vi "Ball ROI (SubVI).vi"(5 "ROI Descriptor COLOR Mask":T2={"Global Rectangle"=[109, 72, 345, 284], "Contours"=[{"ID"=enum."External", "Type"=3, "Coordinates"=[109, 72, 345, 284]}]} {"Contours"."Type" items=["No Selection", "Point", "Line", "Rectangle", "Oval", "Polygon", "Freehand Region", "Annulus", "Unused2", "Unused3", "Broken Line", "Freehand Line", "Rotated Rectangle"]}, 6 "divider (circle)":dbl=1.0, 8 "curY":dbl, 9 "curX":dbl, 10 "Boolean":bool, 11 "Digital in":refnum<vi>) -> (0 "x1":i32, 1 "y0":i32, 2 "x0":i32, 3 "ROI Descriptor COLOR Mask out":T2={"Global Rectangle"=[109, 72, 345, 284], "Contours"=[{"ID"=enum."External", "Type"=3, "Coordinates"=[109, 72, 345, 284]}]} {"Contours"."Type" items=["No Selection", "Point", "Line", "Rectangle", "Oval", "Polygon", "Freehand Region", "Annulus", "Unused2", "Unused3", "Broken Line", "Freehand Line", "Rotated Rectangle"]}, 4 "y1":i32)   [LabVIEW 2017]
panel:
  out "output cluster":T1
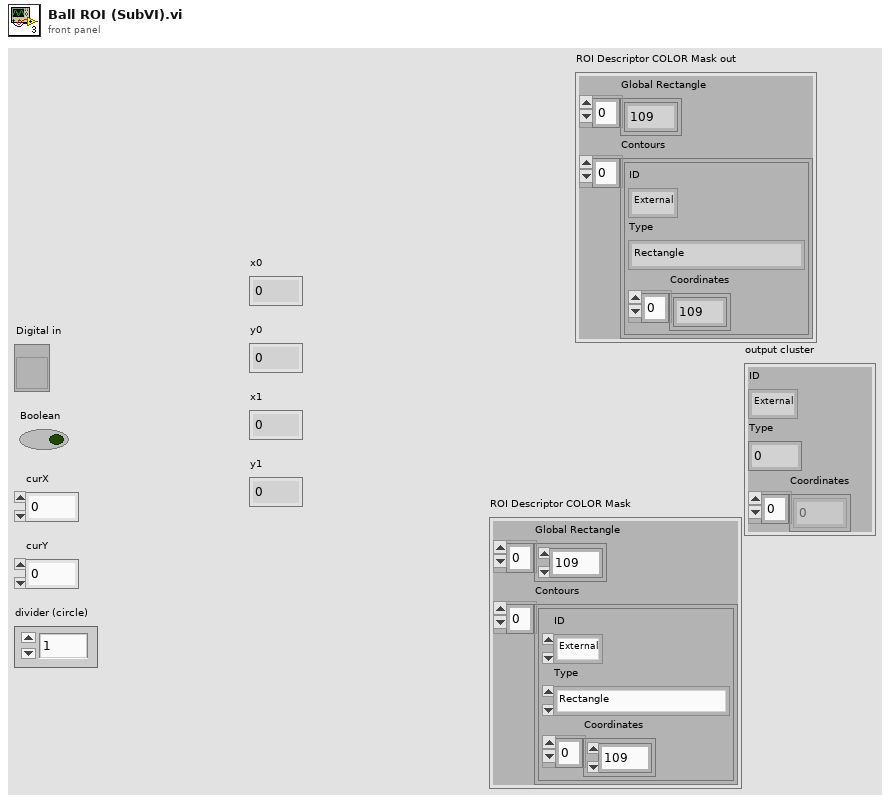
[diagram p1: front panel]
types:
  T1 = cluster{"ID":enum32{"External", "Internal"}, "Type":u32, "Coordinates":i32[]}
  T2 = cluster{"Global Rectangle":i32[], "Contours":cluster{"ID":enum32{"External", "Internal"}, "Type":u32, "Coordinates":i32[]}[]}
  T3 = cluster{"ID":enum32{"External", "Internal"}, "Type":u32, "Coordinates":i32[]}[]
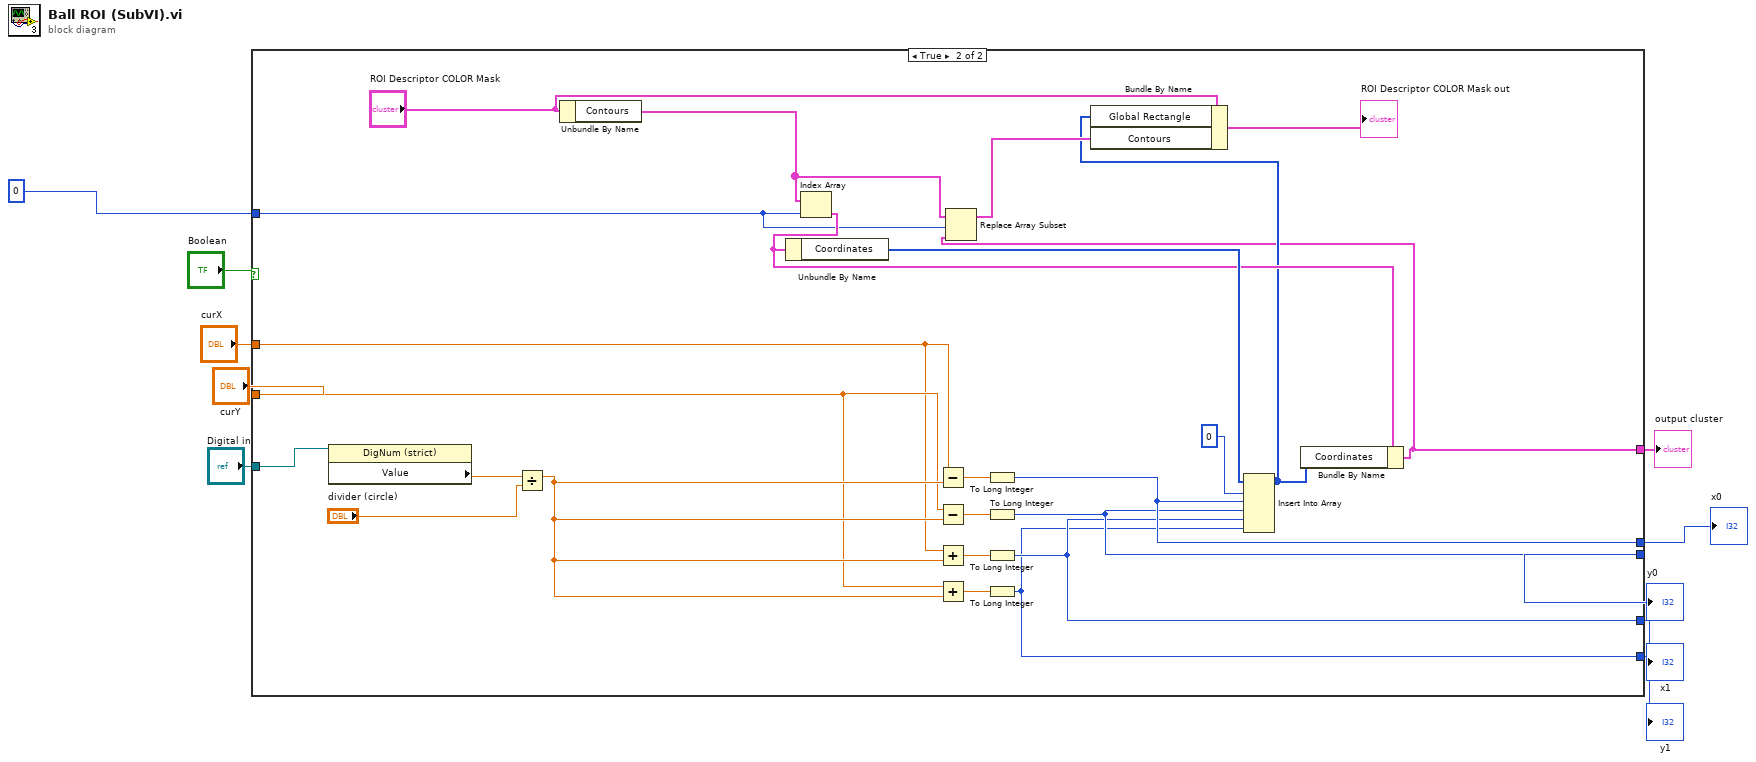
[diagram p0: block diagram]
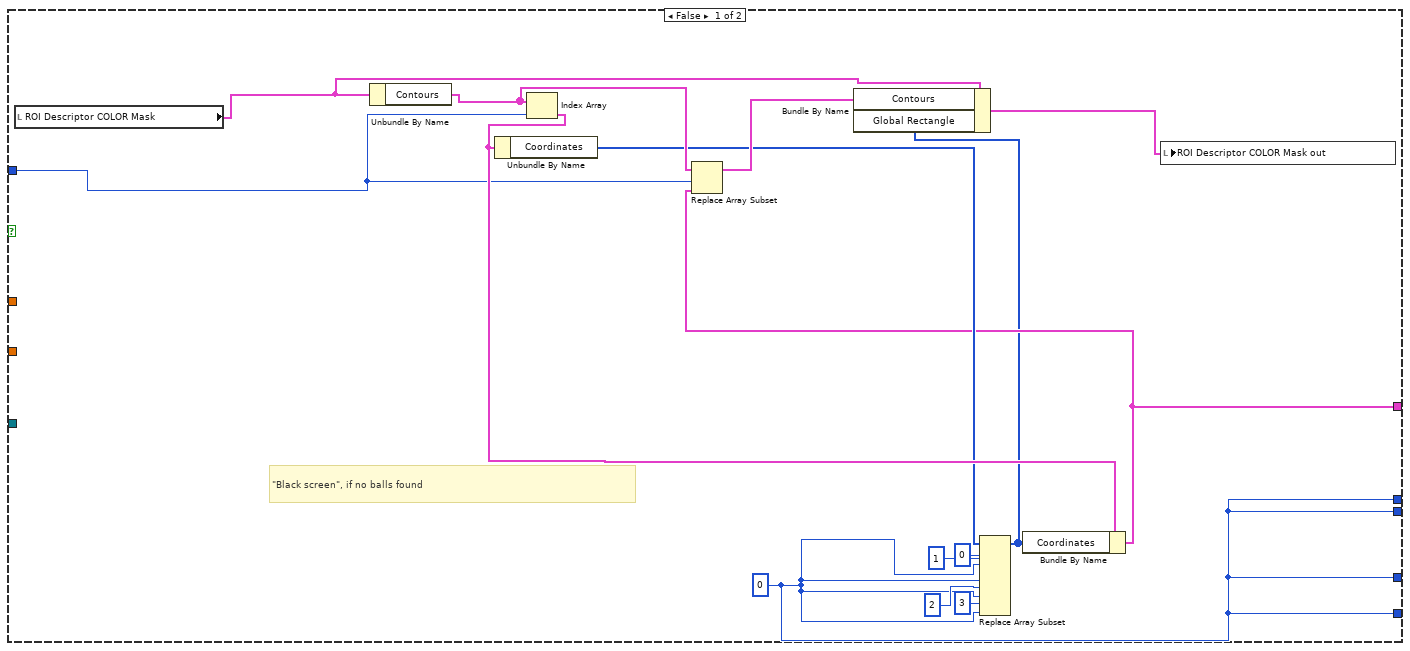
[diagram p2: hidden frame]
diagram:
  n1 = case shown="True" "Boolean" {
    tunnel: 0 ("Ball index") -> [w13 w27]
    tunnel: [w19 w30] -> w5
    tunnel: [w19 w31] -> w6
    tunnel: [w19 w33] -> w7
    tunnel: [w19 w32] -> w8
    tunnel: "curY" -> [_ w39]
    tunnel: "curX" -> [_ w38]
    tunnel: "Digital in" -> [_ w37]
    tunnel: [w12 w26] -> w1
    frame False {
      w19 = 0 ("index")
      # "\"Black screen\", if no balls found"
      n2 = local read "ROI Descriptor COLOR Mask"() -> (w15:T2)
      n3 = Unbundle By Name(w15) -> ("Contours"=w18:T3)
      n4 = Index Array(array=w18, index=w13) -> (element=w17:T1)
      n5 = Unbundle By Name(w17) -> ("Coordinates"=w16:i32[])
      n6 = Replace Array Subset(array=w16, new element #1=w19, index #1=0 ("index"), new element #2=w19, index #2=1 ("index"), new element #3=w19, index #3=2 ("index"), new element #4=w19, index #4=3 ("index")) -> (w11:i32[])
      n7 = Bundle By Name(cluster=w17, "Coordinates"=w11) -> (w12:T1)
      n8 = Replace Array Subset(array=w18, new element=w12, index=w13) -> (w20:T3)
      n9 = Bundle By Name(cluster=w15, "Contours"=w20, "Global Rectangle"=w11) -> (w14:T2)
      n10 = local write "ROI Descriptor COLOR Mask out"(w14) -> ()
    }
    frame True {
      n11 = property class="DigNum (strict)"(reference=w37) -> ("Value"=w40:dbl)  [unwired: 1 in, 2 out]
      n12 = Divide(x=w40, y="divider (circle)") -> (x/y=w44:dbl)
      n13 = Unbundle By Name("ROI Descriptor COLOR Mask") -> ("Contours"=w41:T3)
      n14 = Index Array(array=w41, index=w27) -> (element=w42:T1)
      n15 = Unbundle By Name(w42) -> ("Coordinates"=w43:i32[])
      n16 = Subtract(x=w38, y=w44) -> (x-y=w48:dbl)
      n17 = Subtract(x=w39, y=w44) -> (x-y=w47:dbl)
      n18 = Add(x=w38, y=w44) -> (x+y=w45:dbl)
      n19 = Add(x=w39, y=w44) -> (x+y=w46:dbl)
      n20 = To Long Integer(number=w48) -> (32bit integer=w33:i32)
      n21 = To Long Integer(number=w47) -> (32bit integer=w32:i32)
      n22 = To Long Integer(number=w45) -> (32bit integer=w31:i32)
      n23 = To Long Integer(number=w46) -> (32bit integer=w30:i32)
      n24 = Insert Into Array(array=w43, index=0, new element #1=w33, new element #2=w32, new element #3=w31, new element #4=w30) -> (w28:i32[])
      n25 = Bundle By Name(cluster=w42, "Coordinates"=w28) -> (w26:T1)
      n26 = Replace Array Subset(array=w41, new element=w26, index=w27) -> (w29:T3)
      n27 = Bundle By Name(cluster="ROI Descriptor COLOR Mask", "Global Rectangle"=w28, "Contours"=w29) -> (→"ROI Descriptor COLOR Mask out":T2)
    }
  }
  "y0" <- w8
  "x0" <- w7
  "x1" <- w6
  "y1" <- w5
  "output cluster" <- w1
